vi "Length.vi"(11 "Dictionary in":variant) -> (3 "Dictionary out":variant, 5 "Length":i32)   [LabVIEW 2013, in "Dictionary.lvlib"]
doc: "Returns the length (number of items) in the dictionary. \n\n*NOTE*\nBe careful not to call this VI if unnecessary as it reads all keys from the dictionariy then does a count of those items."
uses:
  Dictionary.lvlib
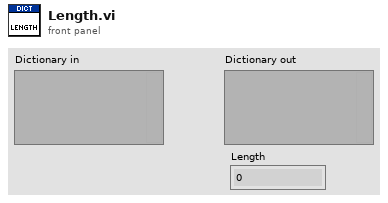
[diagram p1: front panel]
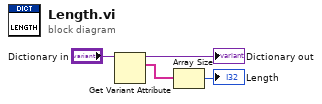
[diagram p0: block diagram]
diagram:
  n1 = Get Variant Attribute(Variant="Dictionary in") -> (duplicate Variant=→"Dictionary out":variant, names=w2:string[])  [unwired: 3 in, 2 out]
  n2 = Array Size(array=w2) -> (size(s)=→"Length":i32)
